vi "3_FM.vi"() -> ()   [LabVIEW 2026]
uses:
  <vilib>/measure/maresamp.llb/Align M + N Waveforms (single shot).vi
  <vilib>/measure/NI_MAPro.lvlib
panel:
  out "message":dynamicdata(graph)
  out "cos carrier":dynamicdata(graph)
  out "Waveform Graph":waveform(dbl)[](graph)
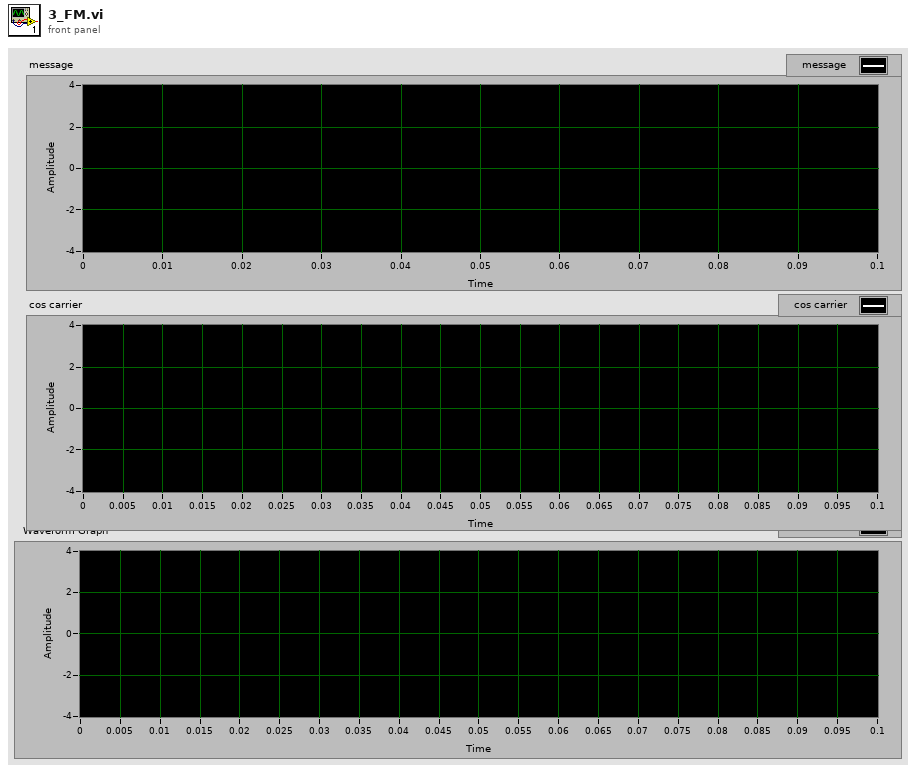
[diagram p1: front panel]
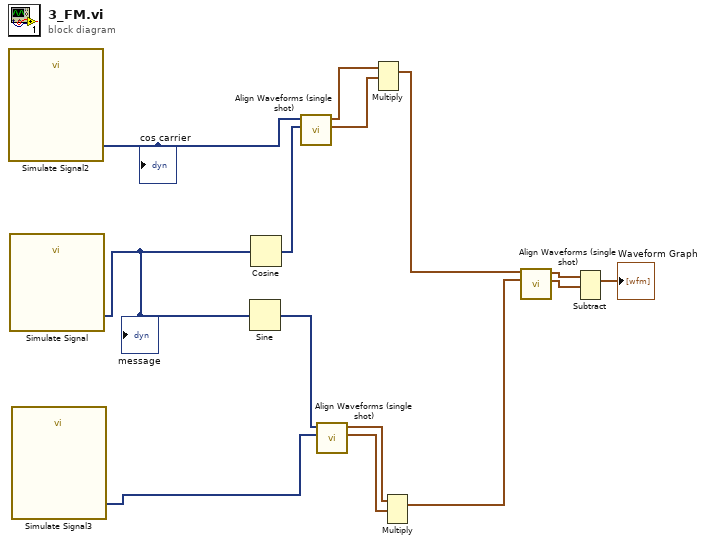
[diagram p0: block diagram]
diagram:
  n1 = call "Simulate Signal2"() -> ("cos carrier"=w13:dynamicdata)  [unwired: 14 in, 1 out]
  "cos carrier" <- w13
  n2 = call "Simulate Signal"() -> ("message"=w5:dynamicdata)  [unwired: 14 in, 1 out]
  "message" <- w5
  n3 = call "Simulate Signal3"() -> ("sin carrier"=w9:dynamicdata)  [unwired: 14 in, 1 out]
  n4 = Sine(x=w5) -> (sin(x)=w8:dynamicdata)
  n5 = Cosine(x=w5) -> (cos(x)=w12:dynamicdata)
  n6 = call-poly <vilib>:"Align Waveforms (single shot).vi"("N waveforms in"=w12, "M waveforms in"=w13) -> ("N aligned waveforms out"=w10:waveform(dbl)[], "M aligned waveforms out"=w11:waveform(dbl)[])  [unwired: 7 in, 1 out]
  n7 = call-poly <vilib>:"Align Waveforms (single shot).vi"("N waveforms in"=w9, "M waveforms in"=w8) -> ("N aligned waveforms out"=w7:waveform(dbl)[], "M aligned waveforms out"=w6:waveform(dbl)[])  [unwired: 7 in, 1 out]
  n8 = Multiply(1:w10, 2:w11) -> (0:w4:waveform(dbl)[])  [unwired: 1 in, 1 out]
  n9 = Multiply(1:w7, 2:w6) -> (0:w3:waveform(dbl)[])  [unwired: 1 in, 1 out]
  n10 = call-poly <vilib>:"Align Waveforms (single shot).vi"("N waveforms in"=w3, "M waveforms in"=w4) -> ("N aligned waveforms out"=w1:waveform(dbl)[], "M aligned waveforms out"=w2:waveform(dbl)[])  [unwired: 7 in, 1 out]
  n11 = Subtract(1:w1, 2:w2) -> (0:→"Waveform Graph":waveform(dbl)[])  [unwired: 1 in, 1 out]
